vi "Lookup Implementor.vi"(8 "error in (no error)":errorcluster, 10 "Implementor ID":string, 11 "Data in":T1) -> (0 "error out":errorcluster, 1 "Found?":bool, 2 "Implementor Full Qualified Name":string, 3 "Data out":T1)   [LabVIEW 2020, in "Peek Window.lvlib"]
uses:
  Peek Window.lvlib
  Open Diagram Argument--cluster.ctl
  MHL Data Cluster.ctl
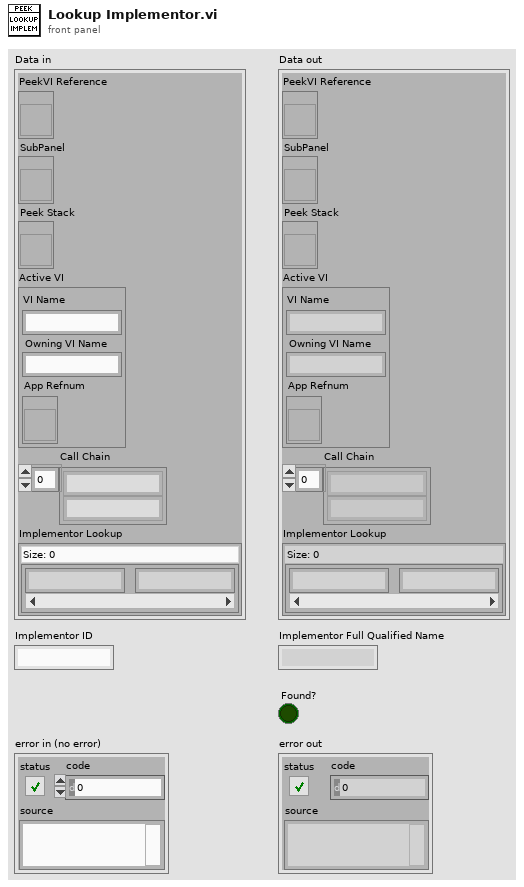
[diagram p1: front panel]
types:
  T1 = typedef "Peek Window.lvlib/MHL Data Cluster.ctl" = cluster{"PeekVI Reference":refnum<vi>, "SubPanel":refnum<vi>, "Peek Stack":refnum<vi>, "Active VI":T2, "Call Chain":string[], "Implementor Lookup":map{string, string}}
  T2 = typedef "Peek Window.lvlib/Open Diagram Argument--cluster.ctl" = cluster{"VI Name":string, "Owning VI Name":string, "App Refnum":refnum<vi>}
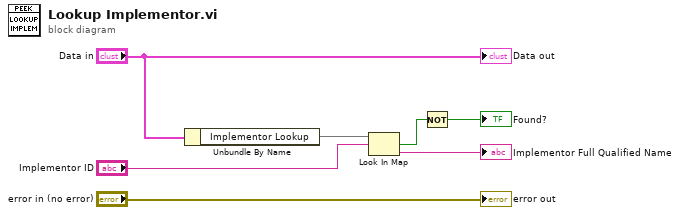
[diagram p0: block diagram]
diagram:
  n1 = Unbundle By Name("Data in") -> ("Implementor Lookup"=w6:map{string, string})
  n2 = Look In Map(map=w6, key="Implementor ID") -> (key not found?=w3:bool, value=→"Implementor Full Qualified Name":string)  [unwired: 1 in]
  n3 = Not(x=w3) -> (.not. x?=→"Found?":bool)
  "Data out" <- "Data in"
  "error out" <- "error in (no error)"
